vi "setBurstMode.vi"(8 "error in (no error)":errorcluster, 10 "Mode":enum16{"Gated", "Triggered"}(ring), 11 "VISA resource name":refnum<visa-resource-name>) -> (0 "error out":errorcluster, 3 "VISA resource name out":refnum<visa-resource-name>)   [LabVIEW 2023, in "Keysight-33500B.lvlib"]
doc: "<b>Author:</b> Wolfgang\n<b>Description:</b>\nTRIGgered: the instrument outputs a waveform for a number of cycles (burst count) each time a\ntrigger is received from the trigger source (TRIGger[1|2]:SOURce).\nGATed: burst count, burst period, and trigger source are ignored (these are used for the triggered\nburst mode only). If a manual trigger is received (TRIGger[1|2] ), it is ignored and no error will be\ngenerated."
uses:
  Keysight-33500B.lvlib
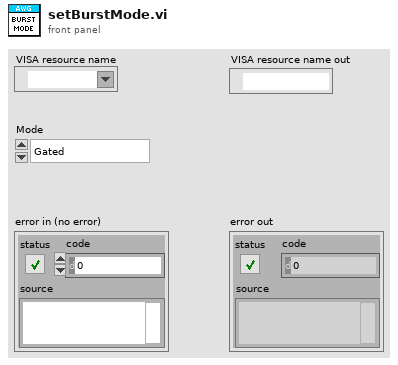
[diagram p1: front panel]
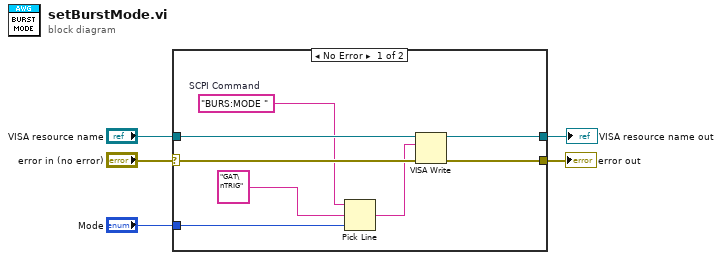
[diagram p0: block diagram]
diagram:
  n1 = case shown="No Error" "error in (no error)" {
    selector: "error in (no error)" -> [w10 w15]
    tunnel: [w12 w14] -> w5
    tunnel: [w13 w15] -> w3
    tunnel: "VISA resource name" -> [w11 w14]
    tunnel: "Mode" -> [w9 _]
    frame No Error {
      w8 = "BURS:MODE "  # SCPI Command
      n2 = Pick Line(string ("")=w8, multi-line string="GAT\nTRIG", line index=w9) -> (output string=w7:string)
      n3 = VISA Write(VISA resource name=w11, write buffer=w7, error in (no error)=w10) -> (VISA resource name out=w12:refnum<visa-resource-name>, error out=w13:errorcluster)  [unwired: 1 out]
    }
    frame Error {
    }
  }
  "VISA resource name out" <- w5
  "error out" <- w3
